vi "AD Adaptive Diagnostics.vi"(8 "error in (no error)":errorcluster) -> ()   [LabVIEW 2019]
uses:
  AD Status.ctl
  System Status.ctl
  <vilib>/Rock Robotics/WPI/ThirdParty/REV Robotics/SPARK MAX/Typedef/Spark MAX Idle Mode.ctl
  <vilib>/Rock Robotics/WPI/ThirdParty/REV Robotics/SPARK MAX/Typedef/Spark MAX Control Type.ctl
  <vilib>/Rock Robotics/Network Tables/NT Write Number.vi
  <vilib>/Rock Robotics/Network Tables/NT Write Boolean.vi
  2020 Robot/Framework/Robot Global Data.vi
  <vilib>/Rock Robotics/Network Tables/NT Read Number.vi
  <vilib>/Rock Robotics/Network Tables/NT Write String.vi
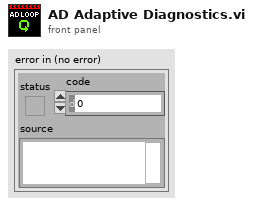
[diagram p1: front panel]
types:
  T1 = typedef "System Status.ctl" = enum16{"System Stable", "LV1", "LV2", "LV3"}
  T2 = typedef "AD Status.ctl" = enum16{"Starting up", "Active", "Transfering Data", "Done"}
  T3 = enum16{"open", "replace", "create", "open or create", "replace or create", "replace or create with confirmation"}
  T4 = typedef "Spark MAX Control Type.ctl" = enum16{"Percent VBus", "Voltage", "Velocity", "Position", "Smart Motion", "Current", "Smart Velocity"}
  T5 = typedef "Spark MAX Idle Mode.ctl" = enum16{"Coast", "Brake"}
  T6 = typedef "ADIS16448 Device Reference.ctl" = cluster{"DevStatus":errorcluster, "Hardware Config":T7, "Calibration Complete":refnum<notifier>, "Last Value Reference":refnum<data-value>, "Sychronous Process VI":T11, "Cmd FIFO":refnum<k33>, "Source":T12, "IMU Status LED Pin":T9, "Calibration Time":u32}
  T7 = typedef "ADIS16448 Hardware Configuration.ctl" = cluster{"SPI Clock Rate (Hz)":dbl, "IMU SPI Mode (3)":T8, "IMU Reset Pin":T9, "IMU SPI Bus":T10, "IMU Data Ready Pin":T9, "Stall Config":cluster{"Pow2BytesPerRead":u8, "StallTicks":u16, "CsToSclkTicks":u8}, "IMU Status LED Pin":T9}
  T8 = typedef "WPI_SPIMode.ctl" = enum16{"Mode 0 (Clk Idle Low,Sample on Leading)", "Mode 1 (Clk Idle Low,Sample on Trailing)", "Mode 2 (Clk Idle High,Sample on Leading)", "Mode 3 (Clk Idle High,Sample on Trailing)"}
  T9 = typedef "FPGA_DIOChannel.ctl" = enum8{"DIO 0", "DIO 1", "DIO 2", "DIO 3", "DIO 4", "DIO 5", "DIO 6", "DIO 7", "DIO 8", "DIO 9", "DIO MXP 0", "DIO MXP 1", "DIO MXP 2", "DIO MXP 3", "DIO MXP 4", "DIO MXP 5", "DIO MXP 6", "DIO MXP 7", "DIO MXP 8", "DIO MXP 9", "DIO MXP 10", "DIO MXP 11", "DIO MXP 12", "DIO MXP 13", "DIO MXP 14", "DIO MXP 15", "SPI Port CS1", "SPI Port CS2", "SPI Port CS3", "SPI Port MISO", "SPI Port MOSI", "Invalid"}
  T10 = typedef "spi_bus.ctl" = enum16{"SPI On-Board, CS0", "SPI On-Board, CS1", "SPI On-Board, CS2", "SPI On-Board, CS3", "SPI MXP", "Invalid"}
  T11 = typedef "ADIS16448 Process.ctl" = refnum<vi>
  T12 = typedef "FPGA_CounterEncoderSourceConvertionLVSourceType.ctl" = cluster{"DevStatus":errorcluster, "AnalogTriggerMode?":bool, "DigitalMode":cluster{"DIO Channel":T13}, "AnalogTriggerMode":cluster{"AnalogTriggerIndex":T14, "OutputType":T15}}
  T13 = typedef "FPGA_DIODigitalSourceChannel.ctl" = enum8{"DIO 0", "DIO 1", "DIO 2", "DIO 3", "DIO 4", "DIO 5", "DIO 6", "DIO 7", "DIO 8", "DIO 9", "DIO MXP 0", "DIO MXP 1", "DIO MXP 2", "DIO MXP 3", "DIO MXP 4", "DIO MXP 5", "DIO MXP 6", "DIO MXP 7", "DIO MXP 8", "DIO MXP 9", "DIO MXP 10", "DIO MXP 11", "DIO MXP 12", "DIO MXP 13", "DIO MXP 14", "DIO MXP 15", "SPI Port CS1", "SPI Port CS2", "SPI Port CS3", "SPI Port MISO", "SPI Port MOSI", "Disabled"}
  T14 = typedef "FPGA_AnalogTriggerIndex.ctl" = enum8{"Trig 0", "Trig 1", "Trig 2", "Trig 3", "Trig 4", "Trig 5", "Trig 6", "Trig 7", "Invalid"}
  T15 = typedef "FPGA_AnalogTriggerOutType.ctl" = enum16{"InWindow", "TriggerState", "Rising", "Falling"}
  T16 = typedef "WPI_MotorControlDeviceRef.ctl" = cluster{"DeviceStatus":errorcluster, "Type":T17, "PWM":cluster{"PWM Channel":T18, "DeadBand":T19}, "CAN":cluster{"Device Number":u8, "SetOutput VI Ref":variant, "GetOutput VI Ref":variant, "Enable VI Ref":variant, "Disable VI Ref":variant, "Data":variant}, "Invert":bool, "DIO PWM":cluster{"PWM \"Enable\" Channel":T18, "DIOChannel":T9, "PWM Rate":dbl}}
  T17 = typedef "WPI_MotorControlType.ctl" = enum16{"PWM", "CAN", "DIO PWM"}
  T18 = typedef "FPGA_DIOPWMChannel.ctl" = enum8{"PWM 0", "PWM 1", "PWM 2", "PWM 3", "PWM 4", "PWM 5", "PWM 6", "PWM 7", "PWM 8", "PWM 9", "PWM MXP 0", "PWM MXP 1", "PWM MXP 2", "PWM MXP 3", "PWM MXP 4", "PWM MXP 5", "PWM MXP 6", "PWM MXP 7", "PWM MXP 8", "PWM MXP 9", "Invalid"}
  T19 = typedef "WPI_PWMDeadband.ctl" = cluster{"Name":string, "maxPositivePwm":i32, "minPositivePwm":i32, "centerPwm":i32, "maxNegativePwm":i32, "minNegativePwm":i32, "angularRange":u16}
  T20 = typedef "ADIS16448 Data.ctl" = cluster{"XAngle":dbl, "YAngle":dbl, "ZAngle":dbl}
  T21 = typedef "ADIS16448 Status.ctl" = cluster{"Calibrated?":bool, "IMU Detected?":bool}
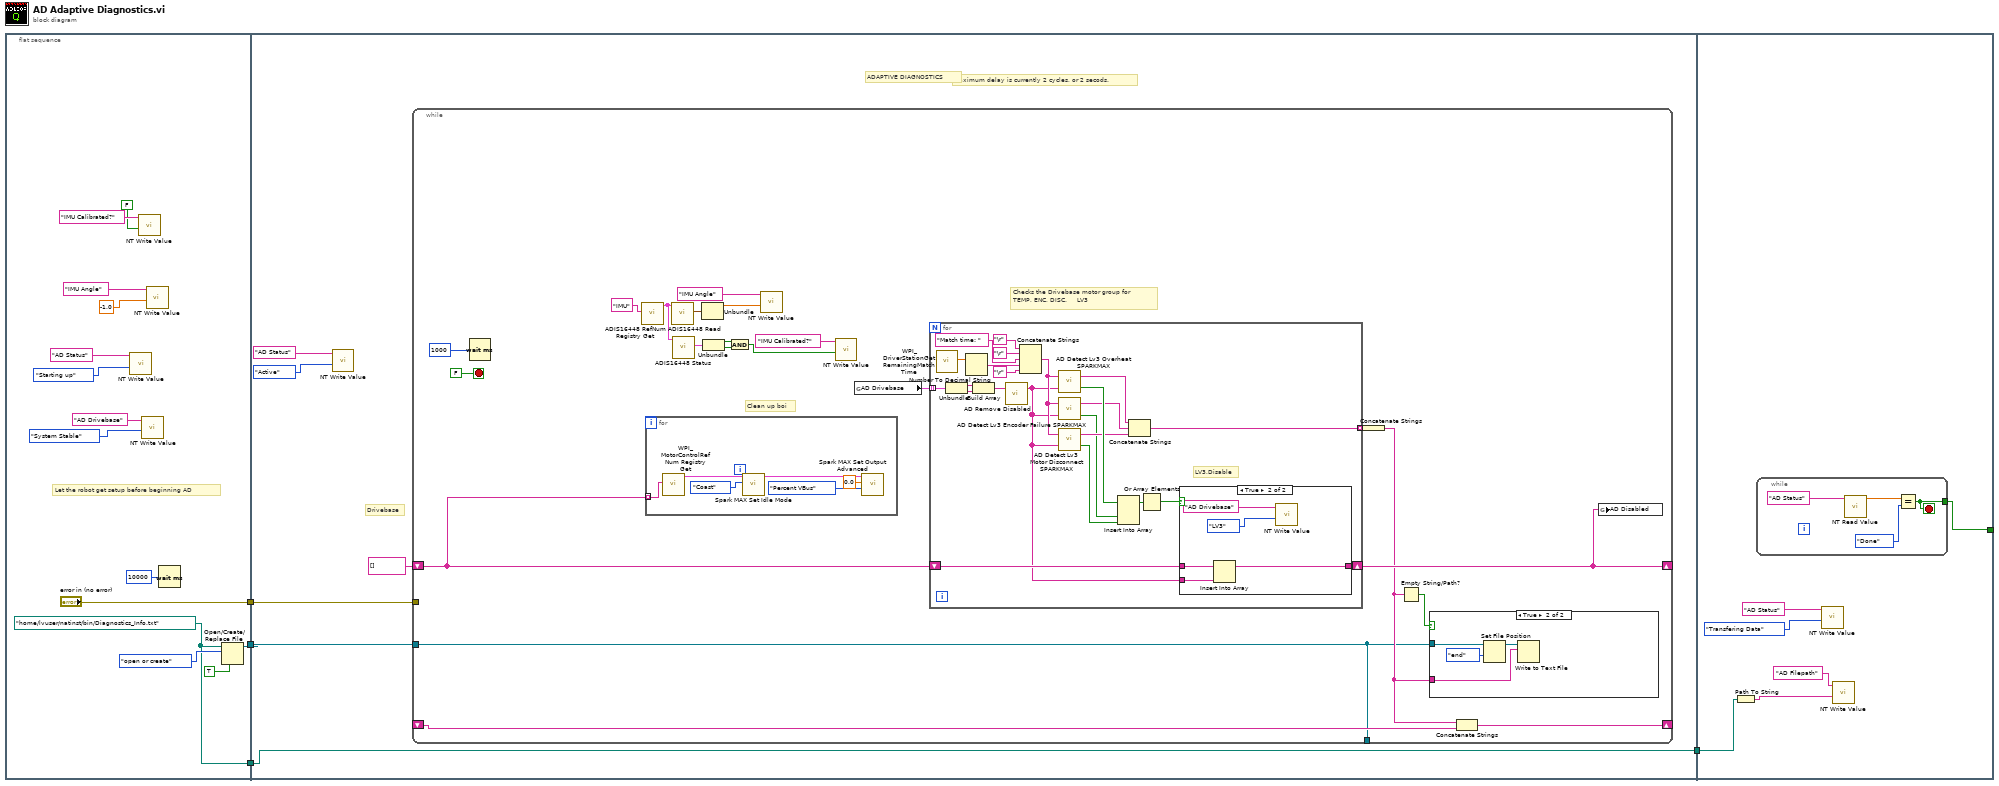
[diagram p0: block diagram]
diagram:
  n1 = flat-sequence {
    tunnel: [w15] -> w4
    tunnel: ["error in (no error)"] -> w3
    tunnel: [w5] -> w2
    tunnel: w4 -> [w20]
    tunnel: w3 -> [w23]
    tunnel: w2 -> [w19]
    tunnel: [w19] -> w1
    tunnel: w1 -> [w86]
    tunnel: [w85] -> _
    frame #0 {
      w5 = path "/home/lvuser/natinst/bin/Diagnostics_Info.txt" ("file path (use dialog)")
      # "Let the robot get setup before beginning AD"
      n2 = call-poly <vilib>:"NT Write Value.vi"("Numeric"=AD_Status."Starting up", "Name"="AD Status") -> ()  [unwired: 9 in, 1 out]
      n3 = call-poly <vilib>:"NT Write Value.vi"("Boolean"=FALSE, "Name"="IMU Calibrated?") -> ()  [unwired: 9 in, 1 out]
      n4 = call-poly <vilib>:"NT Write Value.vi"("Numeric"=System_Status."System Stable" ("Enum"), "Name"="AD Drivebase") -> ()  [unwired: 9 in, 1 out]
      n5 = call-poly <vilib>:"NT Write Value.vi"("Numeric"=-1.0, "Name"="IMU Angle") -> ()  [unwired: 9 in, 1 out]
      n6 = Wait (ms)(milliseconds to wait=u32 10000) -> ()  [unwired: 1 out]
      n7 = Open/Create/Replace File(file path (use dialog)=w5, operation (0:open)=T3."open or create", disable buffering (F)=TRUE) -> (refnum out=w15:refnum<file>)  [unwired: 3 in, 2 out]
    }
    frame #1 {
      # "Maximum delay is currently 2 cycles, or 2 secods."
      # "ADAPTIVE DIAGNOSTICS"
      # "Drivebase"
      n8 = call-poly <vilib>:"NT Write Value.vi"("Numeric"=AD_Status."Active", "Name"="AD Status") -> ()  [unwired: 9 in, 1 out]
      n9 = while {
        shift-right: [w42] -> _
        shift-left: string[] [] -> [w41]
        tunnel: w23 -> [_]
        tunnel: w20 -> [w26]
        shift-right: [w38] -> _
        shift-left: _ -> [w37]
        tunnel: [w26] -> _
        stop <- FALSE stop-if-true
        # "Checks the Drivebase motor group for \nTEMP, ENC, DISC.     LV3"
        # "Clean up boi"
        n10 = Wait (ms)(milliseconds to wait=u32 1000) -> ()  [unwired: 1 out]
        n11 = call "ADIS16448 RefNum Registry Get.vi"("refnum name"="IMU") -> ("ADIS16448DevRef Out"=w28:T6)  [unwired: 9 in, 1 out]
        n12 = for {
          tunnel: w41 -> [w51] mode=indexing
          n13 = call <vilib>:"WPI_MotorControlRefNum Registry Get.vi"("refnum name"=w51) -> ("MotorControlDevRef"=w50:T16)  [unwired: 9 in, 1 out]
          n14 = call <vilib>:"Spark MAX Set Idle Mode.vi"("Idle Mode"=Spark_MAX_Idle_Mode."Coast", "MotorControlDeviceRef in"=w50) -> ("MotorControlDeviceRef out"=w48:T16)  [unwired: 8 in, 1 out]
          n15 = call <vilib>:"Spark MAX Set Output Advanced.vi"("Control Mode"=Spark_MAX_Control_Type."Percent VBus", "Setpoint"=0.0, "MotorControlDevRef"=w48) -> ()  [unwired: 7 in, 2 out]
        }
        n16 = call "ADIS16448 Read.vi"("ADIS16448DevRef"=w28) -> ("Gyro Value"=w33:T20)  [unwired: 3 in, 7 out]
        n17 = call "ADIS16448 Status.vi"("ADIS16448DevRef"=w28) -> ("ADIS16448 Status"=w31:T21)  [unwired: 7 in, 3 out]
        n18 = Unbundle(w33) -> ("XAngle"=w25:dbl)  [unwired: 2 out]
        n19 = Unbundle(w31) -> ("Calibrated?"=w30:bool, "IMU Detected?"=w29:bool)
        n20 = And(x=w30, y=w29) -> (x .and. y?=w27:bool)
        n21 = call-poly <vilib>:"NT Write Value.vi"("Numeric"=w25, "Name"="IMU Angle") -> ()  [unwired: 9 in, 1 out]
        n22 = call-poly <vilib>:"NT Write Value.vi"("Boolean"=w27, "Name"="IMU Calibrated?") -> ()  [unwired: 9 in, 1 out]
        n23 = global read "Robot Global Data.vi" "AD Drivebase"() -> (w43:cluster{"Right":string, "Left":string}[])
        n24 = for {
          tunnel: w43 -> [w70] mode=indexing
          shift-right: [w74] -> w42
          shift-left: w41 -> [w73]
          tunnel: [w61] -> w40 mode=indexing
          # "LV3,Disable"
          n25 = call <vilib>:"WPI_DriverStationGetRemainingMatchTime.vi"() -> ("Match Time(s)"=w66:sgl)  [unwired: 10 in, 1 out]
          n26 = Unbundle(w70) -> ("Right"=w72:string, "Left"=w71:string)
          n27 = Number To Decimal String(number=w66) -> (decimal integer string=w65:string)  [unwired: 1 in]
          n28 = Build Array(w72, w71) -> (w67:string[])
          n29 = call "AD Remove Disabled.vi"("Items In"=w67) -> ("Items Out"=w54:string[])  [unwired: 1 in, 1 out]
          n30 = Concatenate Strings("\r", "\r", "Match time: ", w65, "\r") -> (w55:string)
          n31 = call "AD Detect Lv3 Overheat SPARKMAX.vi"("Motors to test"=w54, "Timing String"=w55) -> ("Disable Motors?"=w58:bool[], "Error Strings"=w59:string[])
          n32 = call "AD Detect Lv3 Encoder Failure SPARKMAX.vi"("Items Out"=w54, "String"=w55) -> ("Array 2"=w52:bool[], "Array"=w53:string[])
          n33 = call "AD Detect Lv3 Motor Disconnect SPARKMAX.vi"("Items Out"=w54, "String"=w55) -> ("Array 2"=w56:bool[], "Array"=w57:string[])
          n34 = Insert Into Array(array=w58, new element #1=w52, new element #2=w56) -> (w69:bool[])  [unwired: 1 in]
          n35 = Concatenate Strings(w59, w53, w57) -> (w61:string)
          n36 = Or Array Elements(Boolean array=w69) -> (logical OR=w68:bool)
          n37 = case shown="True" w68 {
            tunnel: w73 -> [w75 w80]
            tunnel: w54 -> [_ w79]
            tunnel: [w75 w78] -> w74
            frame False {
            }
            frame True {
              n38 = Insert Into Array(array=w80, new element=w79) -> (w78:string[])  [unwired: 1 in]
              n39 = call-poly <vilib>:"NT Write Value.vi"("Numeric"=System_Status."LV3" ("Enum"), "Name"="AD Drivebase") -> ()  [unwired: 9 in, 1 out]
            }
          }
        }
        n40 = Concatenate Strings(w40) -> (w36:string)
        n41 = Empty String/Path?(string/path=w36) -> (empty?=w39:bool)
        n42 = case shown="True" w39 {
          tunnel: w36 -> [_ w84]
          tunnel: w26 -> [_ w81]
          frame False {
          }
          frame True {
            n43 = Set File Position(refnum=w81, from (0:start)=enum16{"start", "end", "current"}."end") -> (refnum out=w83:refnum<file>)  [unwired: 2 in, 1 out]
            n44 = Write to Text File(file (use dialog)=w83, text=w84) -> ()  [unwired: 2 in, 3 out]
          }
        }
        n45 = Concatenate Strings(w36, w37) -> (w38:string)
        n46 = global write "Robot Global Data.vi" "AD Disabled"(w42) -> ()
      }
    }
    frame #2 {
      n47 = Path To String(path=w86) -> (string=w87:string)
      n48 = while {
        tunnel: [w91] -> w85
        stop <- w91 stop-if-true
        n49 = call-poly <vilib>:"NT Read Value.vi"("Name"="AD Status") -> ("Numeric"=w93:dbl)  [unwired: 9 in, 1 out]
        n50 = Equal?(x=w93, y=AD_Status."Done") -> (x = y?=w91:bool)
      }
      n51 = call-poly <vilib>:"NT Write Value.vi"("Numeric"=AD_Status."Transfering Data", "Name"="AD Status") -> ()  [unwired: 9 in, 1 out]
      n52 = call-poly <vilib>:"NT Write Value.vi"("String"=w87, "Name"="AD Filepath") -> ()  [unwired: 9 in, 1 out]
    }
  }
